vi "Set_Tree_Source.vi"(8 "error in (no error)":errorcluster, 10 "data":T1, 11 "IB_SourceTree in":refnum<class "IB_Tree_Source.lvclass">) -> (0 "error out":errorcluster, 3 "IB_SourceTree out":refnum<class "IB_Tree_Source.lvclass">)   [LabVIEW 2020, in "IB_Tree_Source.lvclass"]
uses:
  <vilib>/AppBuilder/IB_Classes/Tree_Source/IB_Tree_Source.lvclass
  <vilib>/AppBuilder/IB_Classes/Tree_Source/IB_Tree_Source.lvclass/IB_Tree_Source.ctl
  <vilib>/AppBuilder/IB_Classes/Tree_Source/IB_Tree_Source.ctl
  <resource>/Framework/Providers/API/ItemRef.ctl
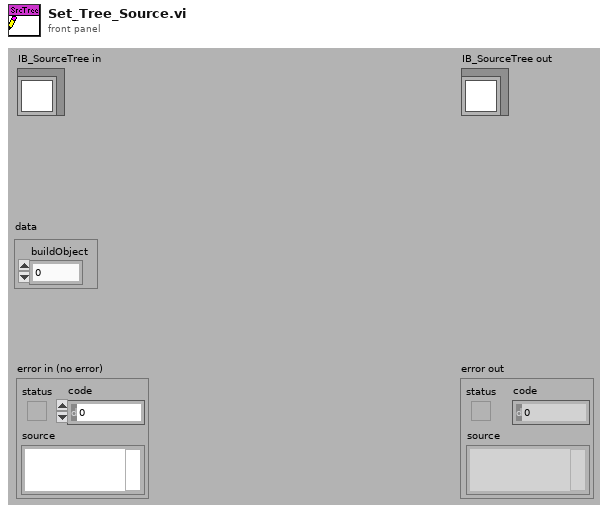
[diagram p1: front panel]
types:
  T1 = typedef "IB_Tree_Source.ctl" = cluster{"buildObject":T2}
  T2 = typedef "ItemRef.ctl" = u64
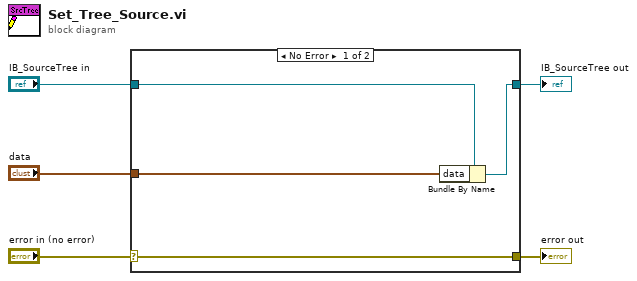
[diagram p0: block diagram]
diagram:
  n1 = case shown="No Error" "error in (no error)" {
    selector: "error in (no error)" -> [w9 w10]
    tunnel: [w9 w10] -> w4
    tunnel: [w7 w11] -> w2
    tunnel: "IB_SourceTree in" -> [w8 w11]
    tunnel: "data" -> [w6 _]
    frame No Error {
      n2 = Bundle By Name(cluster=w8, "data"=w6) -> (w7:refnum<class "IB_Tree_Source.lvclass">)
    }
    frame Error {
    }
  }
  "error out" <- w4
  "IB_SourceTree out" <- w2
